vi "Yale DC Convert.vi"() -> ()   [LabVIEW 2009]
uses:
  QCA Global.vi
panel:
  out "Error":bool
  # "Run this program only when NMR is in Take Data Mode."
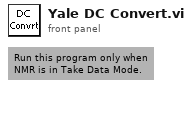
[diagram p1: front panel]
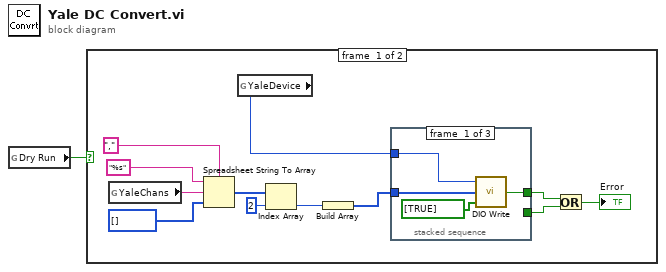
[diagram p0: block diagram]
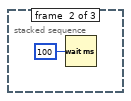
[diagram p2: hidden frame]
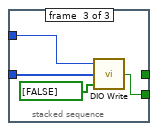
[diagram p3: hidden frame]
diagram:
  n1 = global read "QCA Global.vi" "Dry Run"() -> (w1:bool)
  n2 = case shown="False" w1 {
    frame #0 {
      n3 = global read "QCA Global.vi" "YaleChans"() -> (w10:string)
      n4 = Spreadsheet String To Array(delimiter (Tab)=",", format string="%s", spreadsheet string=w10, array type (2D Dbl)=i32[] [] ("Array Constant")) -> (array=w3:i32[])
      n5 = global read "QCA Global.vi" "YaleDevice"() -> (w9:i16)
      n6 = Index Array(array=w3, index=2 ("Index")) -> (element=w4:i32)
      n7 = Build Array(w4) -> (w5:i32[])
      n8 = stacked-sequence {
        tunnel: w9 -> [w17 _ w22]
        tunnel: w5 -> [w16 _ w21]
        tunnel: [w15 _ _] -> w8
        tunnel: [_ _ w19] -> w7
        frame #0 {
          n9 = call "DIO Write.vi"("Data"=bool[] [TRUE] ("Array Constant"), "Channels"=w16, "device"=w17) -> ("Error"=w15:bool)
        }
        frame #1 {
          n10 = Wait (ms)(milliseconds to wait=u32 100) -> ()  [unwired: 1 out]
        }
        frame #2 {
          n11 = call "DIO Write.vi"("Data"=bool[] [FALSE] ("Array Constant"), "Channels"=w21, "device"=w22) -> ("Error"=w19:bool)
        }
      }
      n12 = Or(x=w8, y=w7) -> (x .or. y?=→"Error":bool)
    }
    frame #1 {
    }
  }
